vi "TestOEPTiming.vi"() -> ()   [LabVIEW 2017]
uses:
  <vilib>/Platform/TimedLoop/XDataNode/timing_clust.ctl
  <vilib>/Platform/TimedLoop/XDataNode/nitl_modes.ctl
  <vilib>/Platform/TimedLoop/XDataNode/wakeup.ctl
  <vilib>/DAQmx/write.llb/DAQmx Write (Analog DBL 1Chan 1Samp).vi
  <vilib>/DAQmx/create/channels.llb/DAQmx Create Channel (AO-Voltage-Basic).vi
  <vilib>/DAQmx/configure/timing.llb/DAQmx Timing (Sample Clock).vi
  <vilib>/DAQmx/miscellaneous.llb/DAQmx Fill In Error Info.vi
  <vilib>/addons/zeromq/zmq_socket.lvclass
  <vilib>/platform/TimedLoop/XDataNode/XDataNode.xnode
  <vilib>/Platform/TimedLoop/XDataNode/XDNodeRunTimeDep.lvlib
  <vilib>/Analysis/NI_AALBase.lvlib
  kernel32.dll
panel:
  out "ts 3":i64
  out "ts 2":i64
  out "ts 1":i64
  in  "Processor":i32=2
  out "ZMQ error":errorcluster
  in  "Start high":bool
  out "OEP-to-LV delay (ms)":T1(graph)
  in  "plot 2 intervals":i32=10
  in  "Loop frequency (Hz)":dbl=5.0
  in  "TTL channel":u16=1 min=1 max=8
  in  "TTL port":u16=5557
  in  "?":bool
  in  "amplitude (V)":dbl=0.05 format="%#_13g"
  in  "AO physical channels":tag="pciDAQ/ao2"
  out "loop error":string=" INSTRUCTIONS:\r\rNormal Use:  When using subVIs that incorporate the error in/error out (or error I/O) structure, place this handler where you want to inform the user of an error, typically at the end of the I/O data path, as the last action of the program.  If the error in error? is ERROR, the handler creates a message describing the error and its source.  If the type of dialog = 1 (default), the message is displayed to the user, who can only acknowedge it.  If the type = 2, the user can acknowledge the message or abort execution; aborting a program with active I/O is not recommended.  If the type = 0, no message is displayed; this is used to process the error programmatically, and the error out cluster elements are wired to individual terminals for that reason.  \r\rOther Use:\n\r\nlocal testing.  To test the error code of a subVI or function that does not have the error I/O structure, you can wire its error code and a source string to the local error code and error source inputs.  If error in error? indicates no error and error code is not equal to 0, the local code and source are substituted for the error in values, and error? is set TRUE (ERROR)."
  in  "plot 1 intervals":i32=10
  out "pulse-to-OEP delay (ms)":T1(graph)
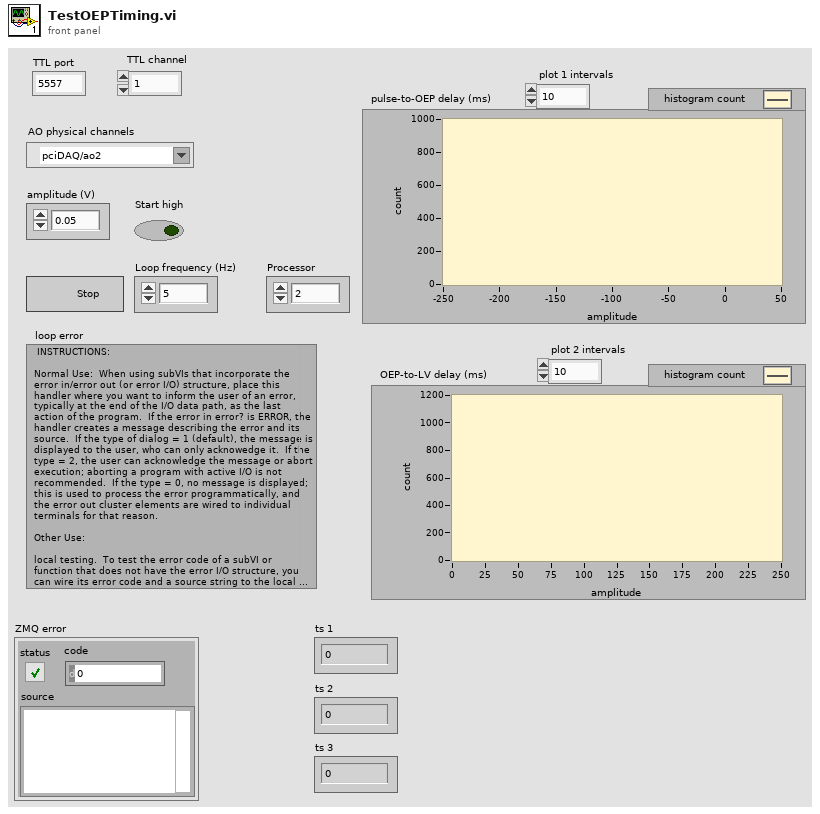
[diagram p1: front panel]
types:
  T1 = cluster{"X Values":dbl[], "Histogram: h(x)":i32[]}
  T2 = typedef "XDNodeRunTimeDep.lvlib/timing_clust.ctl" = cluster{"Expected End [f-1]":u64, "Actual End [f-1]":u64, "Finished Late? [f-1]":bool, "Expected End [i-1]":u64, "Actual End [i-1]":u64, "Finished Late? [i-1]":bool, "Expected Start [i]":u64, "Actual Start [i]":u64, "Expected Start [f]":u64, "Actual Start [f]":u64, "Source Name":string, "Structure Name":string, "Period":i64, "Deadline":i64, "Offset":i64, "Start":i64, "Priority":i32, "Timeout":i32, "Mode":T3, "Wakeup Reason":T4, "Error":errorcluster, "Source Type":string, "Secondary Source Type":string, "Global End Time":u64, "Global Start Time":u64, "Frame Duration":u64, "Iteration Duration":u64, "Assigned CPU":i32, "I/O Scan Engine Mode":u32}
  T3 = typedef "XDNodeRunTimeDep.lvlib/nitl_modes.ctl" = enum32{"No Change", "Process missed periods, maintain original phase", "Discard missed periods, maintain original phase", "Process missed periods, ignore original phase", "Discard missed periods, ignore original phase"}
  T4 = typedef "XDNodeRunTimeDep.lvlib/wakeup.ctl" = enum32{"Normal", "Aborted", "Asynchronous wakeup", "Timing source error", "Timed loop error", "Timeout"}
  T5 = enum16{"big-endian, network order", "native, host order", "little-endian"}
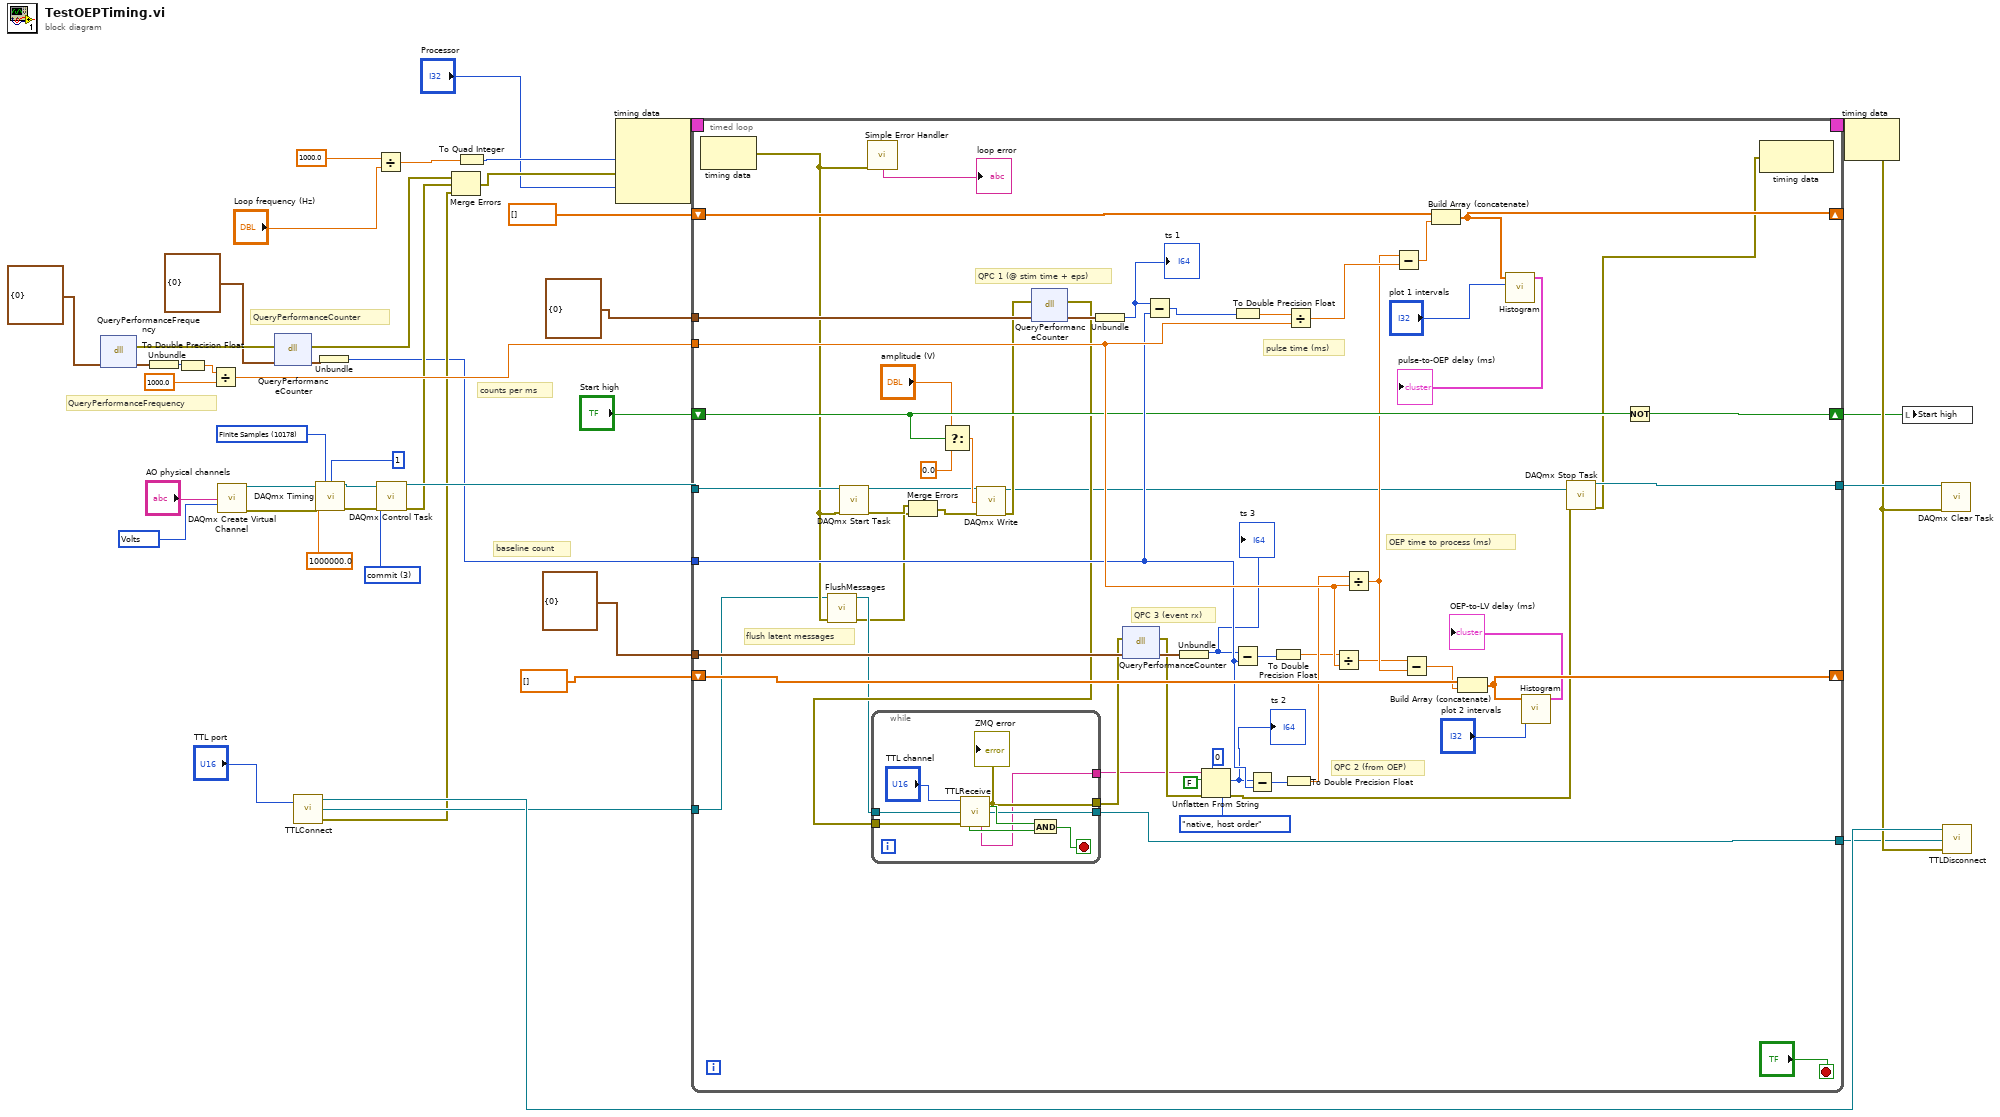
[diagram p0: block diagram]
diagram:
  w9 = 3 items=["verify"=2, "reserve"=4, "commit"=3, "unreserve"=5, "abort"=6] ("action")
  w28 = 10178 items=["Finite Samples"=10178, "Continuous Samples"=10123, "Hardware Timed Single Point"=12522] ("sample mode")
  w39 = 10348 items=["Volts"=10348, "From Custom Scale"=10065] ("units")
  # "QueryPerformanceCounter"
  # "baseline count"
  # "counts per ms"
  # "QueryPerformanceFrequency"
  n1 = dll-call lib="kernel32.dll" fn="QueryPerformanceFrequency"("lpFrequency"=cluster{i64} {0}) -> (error out=w8:errorcluster, "lpFrequency"=w41:cluster{i64})  [unwired: 4 in, 1 out]
  n2 = Unbundle(w41) -> (w23:i64)
  n3 = To Double Precision Float(number=w23) -> (double precision float=w21:dbl)
  n4 = Divide(x=w21, y=1000.0) -> (x/y=w20:dbl)
  n5 = call-poly <vilib>:"DAQmx Create Virtual Channel.vi"("physical channels"="AO physical channels", "units"=w39) -> ("task out"=w24:refnum<k21>, "error out"=w27:errorcluster)  [unwired: 12 in]
  n6 = dll-call lib="kernel32.dll" fn="QueryPerformanceCounter"(error in=w8, cluster{i64} {0}) -> (error out=w6:errorcluster, w4:cluster{i64})  [unwired: 3 in, 1 out]
  n7 = call "TTLConnect.vi"("port"="TTL port") -> ("context out"=w37:refnum<class "zmq_context.lvclass">, "socket out"=w36:refnum<class "zmq_socket.lvclass">, "error out"=w16:errorcluster)  [unwired: 1 in]
  n8 = call-poly <vilib>:"DAQmx Timing.vi"("task/channels in"=w24, "sample mode"=w28, "samples per channel"=1, "rate"=1000000.0, "error in"=w27) -> ("task out"=w19:refnum<k21>, "error out"=w25:errorcluster)  [unwired: 9 in]
  n9 = Unbundle(w4) -> (w5:i64)
  n10 = Divide(x=1000.0, y="Loop frequency (Hz)") -> (x/y=w35:dbl)
  n11 = call <vilib>:"DAQmx Control Task.vi"("task/channels in"=w19, "action"=w9, "error in"=w25) -> ("task out"=w26:refnum<k21>, "error out"=w17:errorcluster)  [unwired: 11 in]
  n12 = Merge Errors(w6, w17, w16) -> (w18:errorcluster)
  n13 = To Quad Integer(1:w35) -> (0:w34:i64)
  n14 = node-c288(w34, w18, "Processor") -> (w44:T2)  [unwired: 1 in]
  n15 = timed-loop {
    timing: w44 -> [_]
    timing-out: [_] -> w43
    shift-right: [w98] -> _
    shift-left: dbl[] [] -> [w100]
    tunnel: w26 -> [w91]
    tunnel: [w90] -> w31
    tunnel: w36 -> [w49]
    tunnel: w20 -> [w94]
    tunnel: cluster{i64} {0} -> [w96]
    tunnel: cluster{i64} {0} -> [w95]
    shift-right: [w92] -> _
    shift-left: dbl[] [] -> [w93]
    tunnel: w5 -> [w89]
    shift-right: [w88] -> w2
    shift-left: "Start high" -> [w87]
    tunnel: [w85] -> w1
    stop <- "?" stop-if-true
    # "flush latent messages"
    # "QPC 3 (event rx)"
    # "OEP time to process (ms)"
    # "QPC 2 (from OEP)"
    # "pulse time (ms)"
    # "QPC 1 (@ stim time + eps)"
    n16 = node-c288() -> (w50:errorcluster)  [unwired: 1 in]
    n17 = call "FlushMessages.vi"("error in (no error)"=w50, "zmq_socket in"=w49) -> ("error out"=w45:errorcluster, "zmq_socket out"=w48:refnum<class "zmq_socket.lvclass">)  [unwired: 8 in]
    n18 = call <vilib>:"DAQmx Start Task.vi"("task/channels in"=w91, "error in"=w50) -> ("task out"=w60:refnum<k21>, "error out"=w46:errorcluster)  [unwired: 12 in]
    n19 = call <vilib>:"Simple Error Handler.vi"("error in (no error)"=w50) -> ("message"=→"loop error":string)  [unwired: 4 in, 4 out]
    n20 = Merge Errors(w46, w45) -> (w47:errorcluster)
    n21 = Select(t="amplitude (V)", s=w87, f=0.0) -> (s? t:f=w73:dbl)
    n22 = call-poly <vilib>:"DAQmx Write.vi"("task/channels in"=w60, "data"=w73, "error in"=w47) -> ("task out"=w59:refnum<k21>, "error out"=w72:errorcluster)  [unwired: 10 in, 1 out]
    n23 = dll-call lib="kernel32.dll" fn="QueryPerformanceCounter"(error in=w72, w96) -> (error out=w61:errorcluster, w82:cluster{i64})  [unwired: 3 in, 1 out]
    n24 = while {
      tunnel: w48 -> [w109]
      tunnel: [w104] -> w85
      tunnel: [w103] -> w70
      tunnel: [w102] -> w54
      tunnel: w61 -> [w101]
      stop <- w107 stop-if-true
      n25 = call "TTLReceive.vi"("channel"="TTL channel", "socket in"=w109, "error in"=w101) -> ("new TTL"=w105:bool, "socket out"=w104:refnum<class "zmq_socket.lvclass">, "event on"=w106:bool, "metadata"=w102:string, "error out"=w103:errorcluster)  [unwired: 6 in, 2 out]
      "ZMQ error" <- w103
      n26 = And(x=w105, y=w106) -> (x .and. y?=w107:bool)
    }
    n27 = Unbundle(w82) -> (w53:i64)
    "ts 1" <- w53
    n28 = dll-call lib="kernel32.dll" fn="QueryPerformanceCounter"(error in=w70, w95) -> (error out=w62:errorcluster, w69:cluster{i64})  [unwired: 3 in, 1 out]
    n29 = Subtract(x=w53, y=w89) -> (x-y=w58:i64)
    n30 = Unbundle(w69) -> (w52:i64)
    "ts 3" <- w52
    n31 = Unflatten From String(type=i64 0, binary string=w54, data includes array or string size? (T)=FALSE, byte order (0:big-endian, network order)=T5."native, host order", error in (no error)=w62) -> (value=w55:i64, error out=w51:errorcluster)  [unwired: 1 out]
    "ts 2" <- w55
    n32 = To Double Precision Float(number=w58) -> (double precision float=w81:dbl)
    n33 = Subtract(x=w52, y=w89) -> (x-y=w57:i64)
    n34 = Subtract(x=w55, y=w89) -> (x-y=w56:i64)
    n35 = To Double Precision Float(number=w57) -> (double precision float=w67:dbl)
    n36 = To Double Precision Float(number=w56) -> (double precision float=w71:dbl)
    n37 = Divide(x=w81, y=w94) -> (x/y=w75:dbl)
    n38 = Divide(x=w67, y=w94) -> (x/y=w66:dbl)
    n39 = Divide(x=w71, y=w94) -> (x/y=w68:dbl)
    n40 = Subtract(x=w68, y=w75) -> (x-y=w74:dbl)
    n41 = Subtract(x=w66, y=w68) -> (x-y=w65:dbl)
    n42 = Build Array (concatenate)(w100, w74) -> (w98:dbl[])
    n43 = Build Array (concatenate)(w93, w65) -> (w92:dbl[])
    n44 = call <vilib>:"Histogram.vi"("intervals"="plot 1 intervals", "X"=w98) -> ("Histogram Graph"=→"pulse-to-OEP delay (ms)":T1)  [unwired: 6 in, 3 out]
    n45 = call <vilib>:"Histogram.vi"("intervals"="plot 2 intervals", "X"=w92) -> ("Histogram Graph"=→"OEP-to-LV delay (ms)":T1)  [unwired: 6 in, 3 out]
    n46 = call <vilib>:"DAQmx Stop Task.vi"("task/channels in"=w59, "error in"=w51) -> ("task out"=w90:refnum<k21>, "error out"=w86:errorcluster)  [unwired: 12 in]
    n47 = Not(x=w87) -> (.not. x?=w88:bool)
    n48 = node-c288(w86) -> ()  [unwired: 1 out]
  }
  n49 = node-c288(w43) -> (w14:errorcluster)
  n50 = local write "Start high"(w2) -> ()
  n51 = call <vilib>:"DAQmx Clear Task.vi"("task in"=w31, "error in"=w14) -> ()  [unwired: 13 in, 1 out]
  n52 = call "TTLDisconnect.vi"("error in"=w14, "socket in"=w1, "context in"=w37) -> ()  [unwired: 1 in, 1 out]
